vi "MCList Adjust.vi"(8 "error in (no error)":errorcluster caption="错误输入（无错误）") -> (0 "error out":errorcluster caption="错误输出")   [LabVIEW 2020]
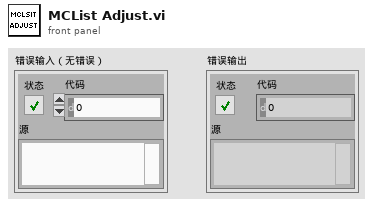
[diagram p1: front panel]
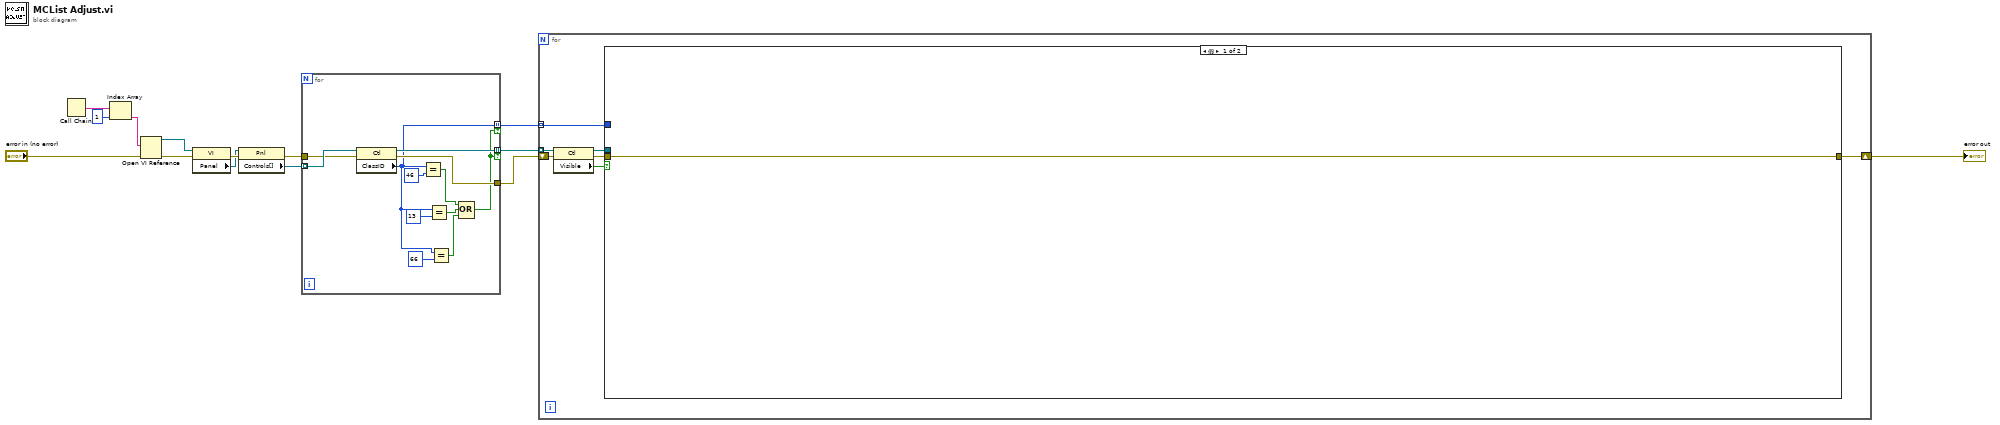
[diagram p0: block diagram]
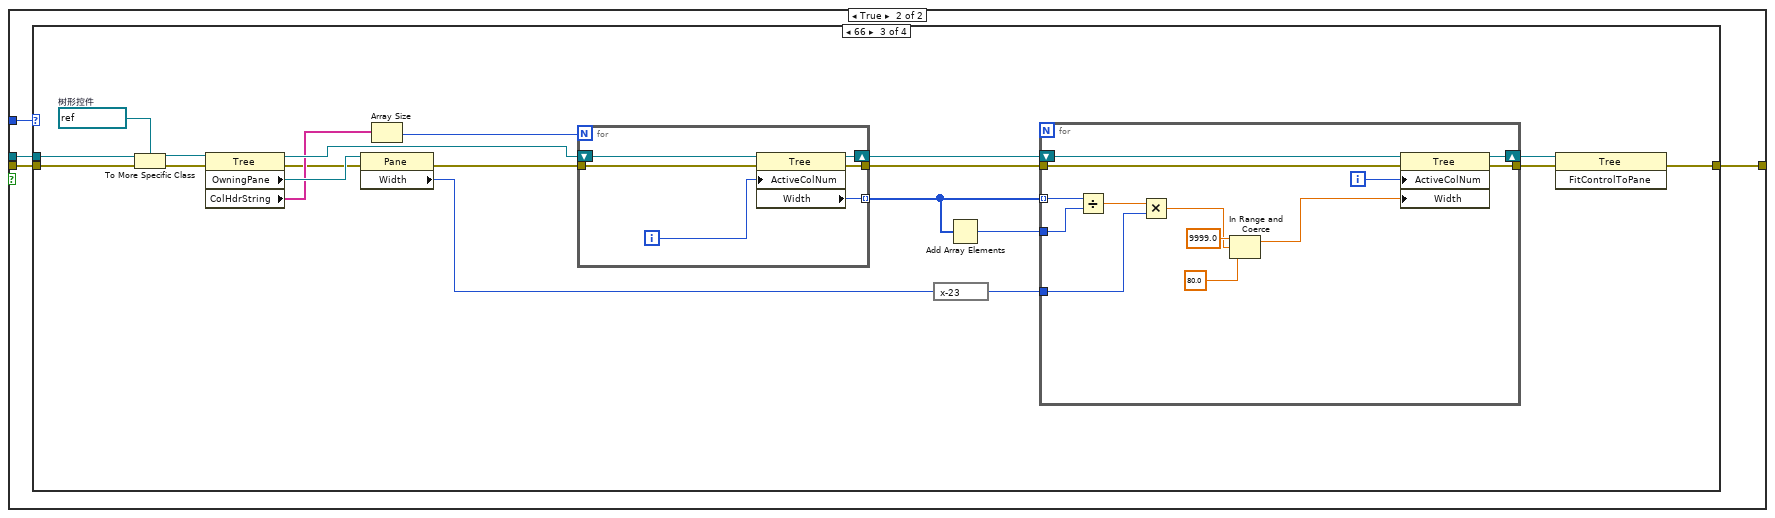
[diagram p2: hidden frame]
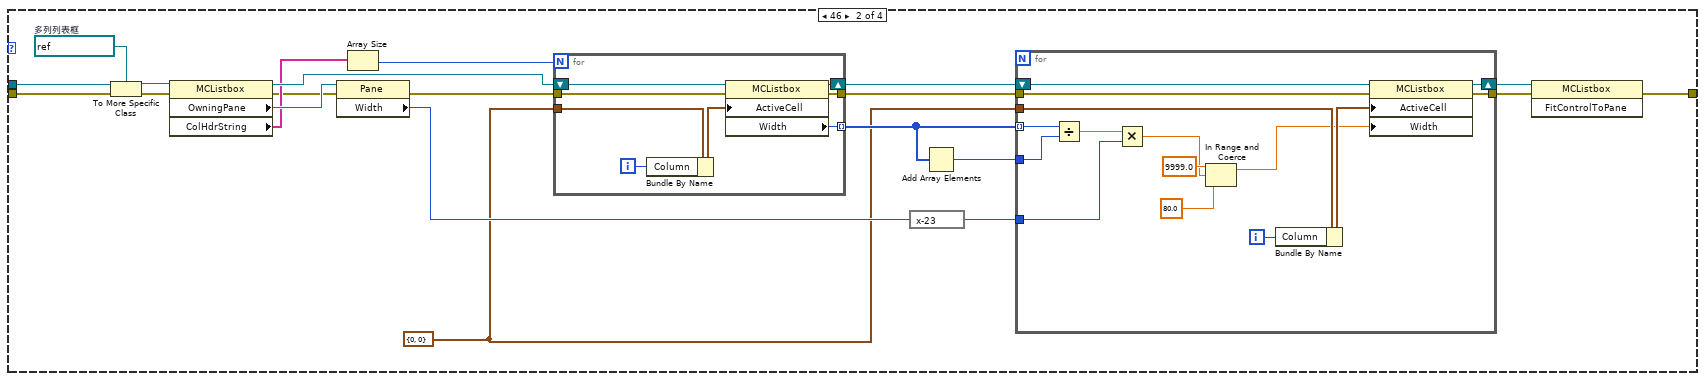
[diagram p4: hidden frame]
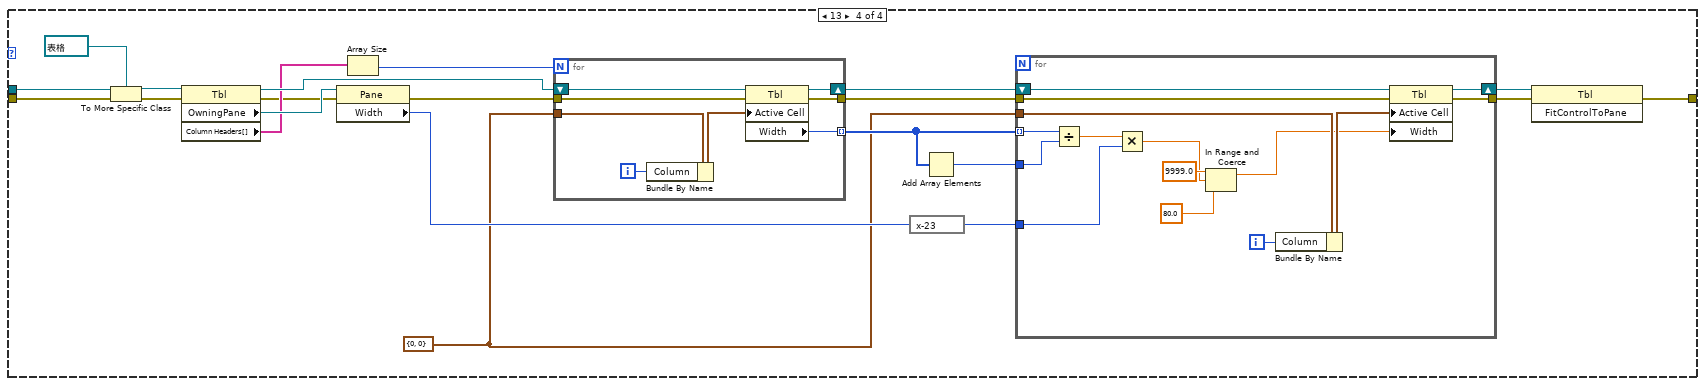
[diagram p5: hidden frame]
diagram:
  n1 = Call Chain() -> (call chain=w2:string[])
  n2 = Index Array(array=w2, index=1 ("索引")) -> (element=w4:string)
  n3 = Open VI Reference(vi path=w4, error in (no error)="error in (no error)") -> (vi reference=w5:refnum<vi>, error out=w10:errorcluster)  [unwired: 4 in]
  n4 = property class="VI"(reference=w5, error in=w10) -> (error out=w11:errorcluster, "Panel"=w6:refnum<vi>)  [unwired: 1 out]
  n5 = property class="Pnl"(reference=w6, error in=w11) -> (error out=w12:errorcluster, "Controls[]"=w7:refnum<vi>[])  [unwired: 1 out]
  n6 = for {
    tunnel: w7 -> [w26] mode=indexing
    tunnel: [w24] -> w8 mode=indexing if=w18
    tunnel: w12 -> [w23]
    tunnel: [w22] -> w13
    tunnel: [w16] -> w1 mode=indexing if=w18
    n7 = property class="Ctl"(reference=w26, error in=w23) -> (reference out=w24:refnum<vi>, error out=w22:errorcluster, "ClassID"=w16:u32)
    n8 = Equal?(x=w16, y=u32 46) -> (x = y?=w20:bool)
    n9 = Equal?(x=w16, y=u32 13) -> (x = y?=w19:bool)
    n10 = Equal?(x=w16, y=u32 66) -> (x = y?=w15:bool)
    n11 = Compound Arithmetic op=OR ("复合运算")(w20, w19, w15) -> (w18:bool)
  }
  n12 = for {
    tunnel: w8 -> [w32] mode=indexing
    shift-right: [w30] -> w14
    shift-left: w13 -> [w31]
    tunnel: w1 -> [w29] mode=indexing
    n13 = property class="Ctl"(reference=w32) -> (reference out=w28:refnum<vi>, "Visible"=w27:bool)  [unwired: 1 in, 1 out]
    n14 = case shown="假" w27 {
      tunnel: w31 -> [w33 w37]
      tunnel: [w33 w36] -> w30
      tunnel: w29 -> [_ w35]
      tunnel: w28 -> [_ w34]
      frame False {
      }
      frame True {
        n15 = case shown="66" w35 {
          tunnel: w34 -> [_ w51 w94 w134]
          tunnel: w37 -> [w38 w47 w91 w131]
          tunnel: [w38 w39 w83 w123] -> w36
          frame 0, Default {
          }
          frame 46 {
            w48 = cluster{"Row":i32, "Column":i32} {"Row"=0, "Column"=0} ("活动单元格:活动单元格")
            w50 = refnum<vi> refnum  # 多列列表框
            n16 = To More Specific Class(target class=w50, reference=w51, error in=w47) -> (specific class reference=w49:refnum<vi>, error out=w46:errorcluster)
            n17 = property class="MCListbox"(reference=w49, error in=w46) -> (reference out=w59:refnum<vi>, error out=w45:errorcluster, "OwningPane"=w58:refnum<vi>, "ColHdrString"=w53:string[])
            n18 = property class="Pane"(reference=w58, error in=w45) -> (error out=w44:errorcluster, "Width"=w54:u32)  [unwired: 1 out]
            n19 = Array Size(array=w53) -> (size(s)=w52:i32)
            n20 = for {
              N: w52 -> [_]
              tunnel: [w79] -> w55 mode=indexing
              tunnel: w48 -> [w77]
              tunnel: w44 -> [w76]
              tunnel: [w75] -> w43
              shift-right: [w78] -> w57
              shift-left: w59 -> [w82]
              i -> [w80]
              n21 = Bundle By Name(cluster=w77, "Column"=w80) -> (w81:cluster{"Row":i32, "Column":i32})
              n22 = property class="MCListbox"(reference=w82, error in=w76, "ActiveCell"=w81) -> (reference out=w78:refnum<vi>, error out=w75:errorcluster, "Width"=w79:u32)
            }
            n23 = expression code="x-23"(w54) -> (w42:u32)
            n24 = Add Array Elements(numeric array=w55) -> (sum=w56:u32)
            n25 = for {
              tunnel: w55 -> [w74] mode=indexing
              tunnel: w56 -> [w73]
              tunnel: w48 -> [w69]
              tunnel: w43 -> [w68]
              tunnel: [w67] -> w40
              tunnel: w42 -> [w65]
              shift-right: [w64] -> w41
              shift-left: w57 -> [w72]
              i -> [w71]
              n26 = Divide(x=w74, y=w73) -> (x/y=w66:dbl)
              n27 = Multiply(x=w66, y=w65) -> (x*y=w61:dbl)
              n28 = In Range and Coerce(upper limit=9999.0 ("上限"), x=w61, lower limit=80.0 ("下限")) -> (coerced(x)=w60:dbl)  [unwired: 1 out]
              n29 = Bundle By Name(cluster=w69, "Column"=w71) -> (w70:cluster{"Row":i32, "Column":i32})
              n30 = property class="MCListbox"(reference=w72, error in=w68, "ActiveCell"=w70, "Width"=w60) -> (reference out=w64:refnum<vi>, error out=w67:errorcluster)
            }
            n31 = invoke class="MCListbox" method="FitControlToPane"(reference=w41, error in=w40) -> (error out=w39:errorcluster)  [unwired: 1 in, 2 out]
          }
          frame 66 {
            w93 = refnum<vi> refnum  # 树形控件
            n32 = To More Specific Class(target class=w93, reference=w94, error in=w91) -> (specific class reference=w92:refnum<vi>, error out=w90:errorcluster)
            n33 = property class="Tree"(reference=w92, error in=w90) -> (reference out=w102:refnum<vi>, error out=w89:errorcluster, "OwningPane"=w101:refnum<vi>, "ColHdrString"=w96:string[])
            n34 = property class="Pane"(reference=w101, error in=w89) -> (error out=w88:errorcluster, "Width"=w97:u32)  [unwired: 1 out]
            n35 = Array Size(array=w96) -> (size(s)=w95:i32)
            n36 = for {
              N: w95 -> [_]
              tunnel: [w120] -> w98 mode=indexing
              tunnel: w88 -> [w118]
              tunnel: [w117] -> w87
              shift-right: [w119] -> w100
              shift-left: w102 -> [w121]
              i -> [w116]
              n37 = property class="Tree"(reference=w121, error in=w118, "ActiveColNum"=w116) -> (reference out=w119:refnum<vi>, error out=w117:errorcluster, "Width"=w120:i32)
            }
            n38 = expression code="x-23"(w97) -> (w86:u32)
            n39 = Add Array Elements(numeric array=w98) -> (sum=w99:i32)
            n40 = for {
              tunnel: w98 -> [w115] mode=indexing
              tunnel: w99 -> [w114]
              tunnel: w87 -> [w112]
              tunnel: [w111] -> w84
              tunnel: w86 -> [w109]
              shift-right: [w108] -> w85
              shift-left: w100 -> [w113]
              i -> [w103]
              n41 = Divide(x=w115, y=w114) -> (x/y=w110:dbl)
              n42 = Multiply(x=w110, y=w109) -> (x*y=w105:dbl)
              n43 = In Range and Coerce(upper limit=9999.0 ("上限"), x=w105, lower limit=80.0 ("下限")) -> (coerced(x)=w104:dbl)  [unwired: 1 out]
              n44 = property class="Tree"(reference=w113, error in=w112, "ActiveColNum"=w103, "Width"=w104) -> (reference out=w108:refnum<vi>, error out=w111:errorcluster)
            }
            n45 = invoke class="Tree" method="FitControlToPane"(reference=w85, error in=w84) -> (error out=w83:errorcluster)  [unwired: 1 in, 2 out]
          }
          frame 13 {
            w132 = cluster{"Row":i32, "Column":i32} {"Row"=0, "Column"=0} ("活动单元格:活动单元格")
            n46 = To More Specific Class(target class=refnum<vi> refnum ("Write"), reference=w134, error in=w131) -> (specific class reference=w133:refnum<vi>, error out=w130:errorcluster)
            n47 = property class="Tbl"(reference=w133, error in=w130) -> (reference out=w142:refnum<vi>, error out=w129:errorcluster, "OwningPane"=w141:refnum<vi>, "Column Headers[]"=w136:string[])
            n48 = property class="Pane"(reference=w141, error in=w129) -> (error out=w128:errorcluster, "Width"=w137:u32)  [unwired: 1 out]
            n49 = Array Size(array=w136) -> (size(s)=w135:i32)
            n50 = for {
              N: w135 -> [_]
              tunnel: [w162] -> w138 mode=indexing
              tunnel: w132 -> [w160]
              tunnel: w128 -> [w159]
              tunnel: [w158] -> w127
              shift-right: [w161] -> w140
              shift-left: w142 -> [w165]
              i -> [w163]
              n51 = Bundle By Name(cluster=w160, "Column"=w163) -> (w164:cluster{"Row":i32, "Column":i32})
              n52 = property class="Tbl"(reference=w165, error in=w159, "Active Cell"=w164) -> (reference out=w161:refnum<vi>, error out=w158:errorcluster, "Width"=w162:u32)
            }
            n53 = expression code="x-23"(w137) -> (w126:u32)
            n54 = Add Array Elements(numeric array=w138) -> (sum=w139:u32)
            n55 = for {
              tunnel: w138 -> [w157] mode=indexing
              tunnel: w139 -> [w156]
              tunnel: w132 -> [w152]
              tunnel: w127 -> [w151]
              tunnel: [w150] -> w124
              tunnel: w126 -> [w148]
              shift-right: [w147] -> w125
              shift-left: w140 -> [w155]
              i -> [w154]
              n56 = Divide(x=w157, y=w156) -> (x/y=w149:dbl)
              n57 = Multiply(x=w149, y=w148) -> (x*y=w144:dbl)
              n58 = In Range and Coerce(upper limit=9999.0 ("上限"), x=w144, lower limit=80.0 ("下限")) -> (coerced(x)=w143:dbl)  [unwired: 1 out]
              n59 = Bundle By Name(cluster=w152, "Column"=w154) -> (w153:cluster{"Row":i32, "Column":i32})
              n60 = property class="Tbl"(reference=w155, error in=w151, "Active Cell"=w153, "Width"=w143) -> (reference out=w147:refnum<vi>, error out=w150:errorcluster)
            }
            n61 = invoke class="Tbl" method="FitControlToPane"(reference=w125, error in=w124) -> (error out=w123:errorcluster)  [unwired: 1 in, 2 out]
          }
        }
      }
    }
  }
  "error out" <- w14
